vi "Global Variables.vi"() -> ()   [LabVIEW 2016]
panel:
  out "Lenkstatus":bool
  out "wurde eingegriffen?":bool
  in  "SETTING PARAMETER:":i32
  in  "si":dbl
  in  "ss":dbl
  # "0: NEIN\n1: JA"
  # "0: DO NOTHING\n1: SET TO HUMAN MODE\n2: ENABLE REGLER\n3: needed on NI side only\n    to first set to human and \n    then to activate REGLER!"
  # "LEnkung ein = 1 Lenkung aus =0"
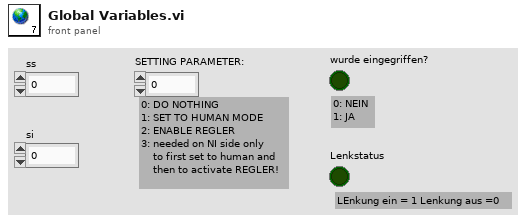
[diagram p1: front panel]
diagram:
